vi "Set VISA Ref.vi"(8 "error in (no error)":errorcluster, 10 "VISA-placeholder":refnum<visa-resource-name>, 11 "Temp01 in":refnum<class "TELLC_Temp01.lvclass">) -> (0 "error out":errorcluster, 3 "Temp01 out":refnum<class "TELLC_Temp01.lvclass">)   [LabVIEW 2017, in "TELLC_Temp01.lvclass"]
doc: "Developed by Kevin Thompson\nkevin@thompsonengineering.net\n\nCopyright 2018\nThompson Engineering, LLC"
uses:
  TELLC_Temp01.lvclass
  TELLC_Temp01.lvclass/TELLC_Temp01.ctl
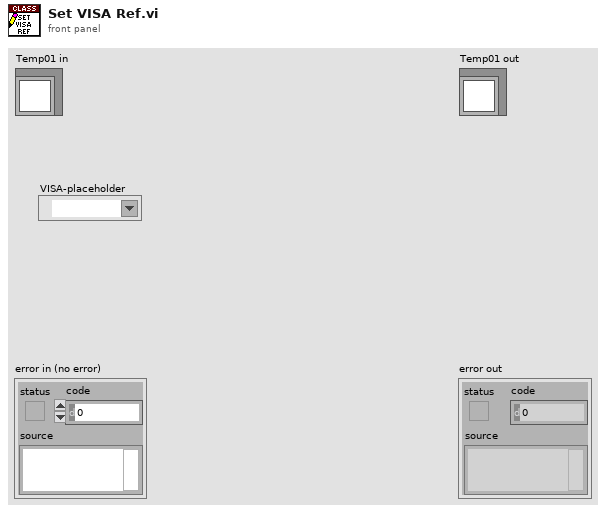
[diagram p1: front panel]
types:
  T1 = typedef "TELLC_Temp01.lvclass/ObjData--cluster.ctl" = cluster{"Settings":T2, "ReadData-placeholder":T3, "VISA-placeholder":refnum<visa-resource-name>}
  T2 = typedef "TELLC_Temp01.lvclass/Settings--cluster.ctl" = cluster{"Simulation":bool}
  T3 = typedef "TELLC_Temp01.lvclass/Read Data--cluster.ctl" = cluster{"Data":dbl}
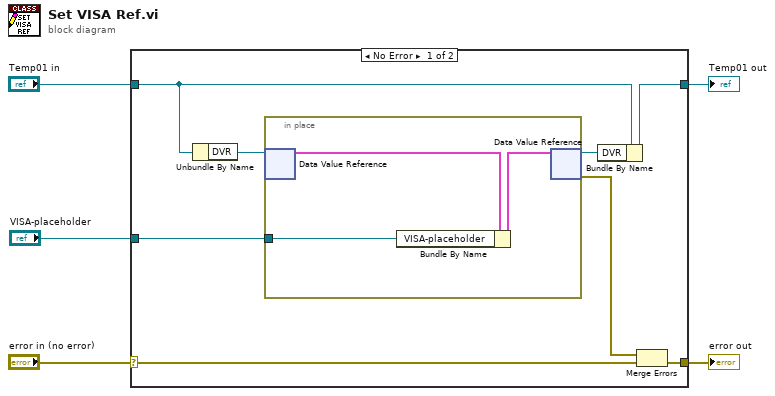
[diagram p0: block diagram]
diagram:
  n1 = case shown="No Error" "error in (no error)" {
    selector: "error in (no error)" -> [w13 w17]
    tunnel: [w7 w17] -> w4
    tunnel: [w9 w18] -> w2
    tunnel: "Temp01 in" -> [w12 w18]
    tunnel: "VISA-placeholder" -> [w8 _]
    frame No Error {
      n2 = Unbundle By Name(w12) -> ("DVR"=w11:refnum<data-value>)
      n3 = in-place {
        in-place-border: w8 -> [w14]
        n4 = in-place-dvr #1(w11) -> (w16:T1)  [unwired: 1 out]
        n5 = Bundle By Name(cluster=w16, "VISA-placeholder"=w14) -> (w15:T1)
        n6 = in-place-dvr #1(w15) -> (w10:refnum<data-value>, w6:errorcluster)
      }
      n7 = Bundle By Name(cluster=w12, "DVR"=w10) -> (w9:refnum<class "TELLC_Temp01.lvclass">)
      n8 = Merge Errors(w6, w13) -> (w7:errorcluster)
    }
    frame Error {
    }
  }
  "error out" <- w4
  "Temp01 out" <- w2
